vi "Eval X-Y-Z(t1,t2).vi"(0 "Start":dbl[](array[numeric])=[0.0, 0.0] format="%.2f", 1 "number of points":u32=25, 2 "End":dbl[](array[numeric])=[1.0, 1.0] format="%.2f", 3 "Formulas":string[](array[string])=["", "", ""], 4 "Variables":string[](array[string])=["t1", "t2"]) -> (5 "X":dbl[](array[numeric]) format="%.2f", 6 "Y":dbl[](array[numeric]) format="%.2f", 7 "Z":dbl[](array[numeric]) format="%.2f", 8 "ticks":u32, 9 "error":i32)   [LabVIEW 2014, in "NI_Gmath.lvlib"]
doc: "Describes a surface in 3D with two variables running over two different intervals."
uses:
  NI_Gmath.lvlib
panel:
  # "Example:\n\n number of points: 25 \n Start: 0.0 and 0.0\n End: 1.0 and 1.0\n Formulas: sin(t1*t2)+t1 and exp(t2) and -t1 \n Variables: t1 and t2"
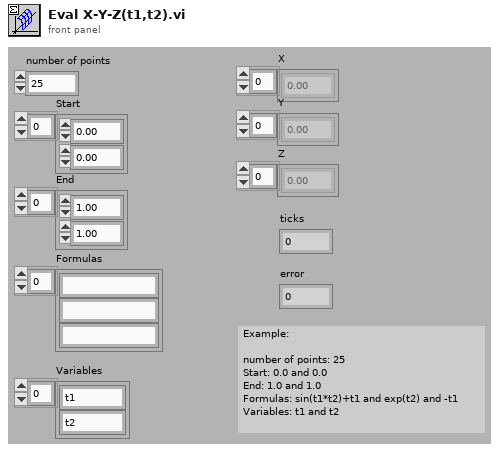
[diagram p1: front panel]
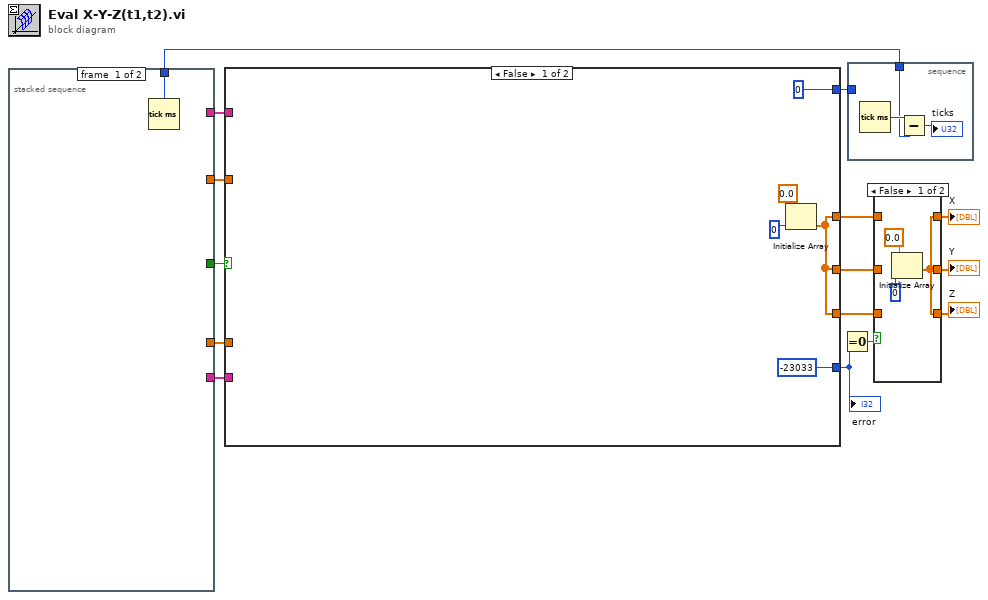
[diagram p0: block diagram]
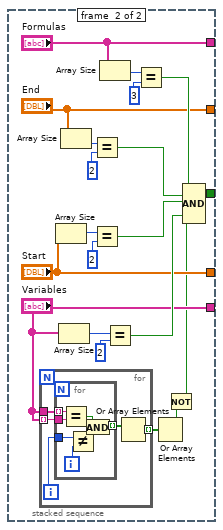
[diagram p3: hidden frame]
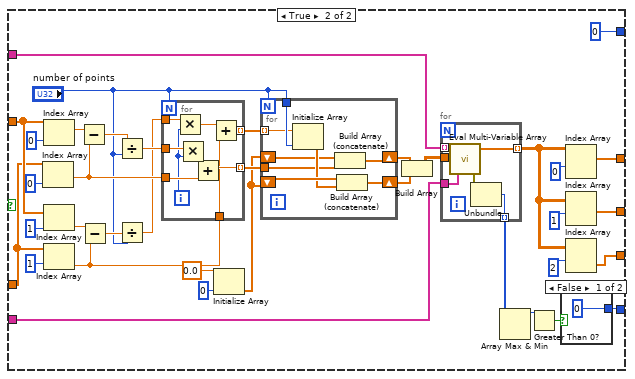
[diagram p4: hidden frame]
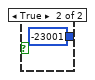
[diagram p5: hidden frame]
diagram:
  n1 = stacked-sequence {
    tunnel: [_ w36] -> w10
    tunnel: [_ "Formulas"] -> w11
    tunnel: [_ "Variables"] -> w12
    tunnel: [_ "Start"] -> w13
    tunnel: [_ "End"] -> w14
    tunnel: [w16 _] -> w9
    frame #0 {
      n2 = Tick Count (ms)() -> (millisecond timer value=w16:u32)
    }
    frame #1 {
      n3 = for {
        tunnel: "Variables" -> [w41]
        tunnel: "Variables" -> [w40] mode=indexing
        tunnel: [w37] -> w21 mode=indexing
        i -> [w39]
        n4 = for {
          tunnel: w41 -> [w48] mode=indexing
          tunnel: w40 -> [w47]
          tunnel: w39 -> [w46]
          tunnel: [w42] -> w38 mode=indexing
          i -> [w45]
          n5 = Equal?(x=w48, y=w47) -> (x = y?=w44:bool)
          n6 = Not Equal?(x=w46, y=w45) -> (x != y?=w43:bool)
          n7 = And(x=w44, y=w43) -> (x .and. y?=w42:bool)
        }
        n8 = Or Array Elements(Boolean array=w38) -> (logical OR=w37:bool)
      }
      n9 = Array Size(array="Start") -> (size(s)=w24:i32)
      n10 = Array Size(array="Variables") -> (size(s)=w28:i32)
      n11 = Array Size(array="End") -> (size(s)=w26:i32)
      n12 = Equal?(x=w26, y=2) -> (x = y?=w33:bool)
      n13 = Equal?(x=w24, y=2) -> (x = y?=w34:bool)
      n14 = Array Size(array="Formulas") -> (size(s)=w30:i32)
      n15 = Equal?(x=w28, y=2) -> (x = y?=w35:bool)
      n16 = Equal?(x=w30, y=3) -> (x = y?=w32:bool)
      n17 = Or Array Elements(Boolean array=w21) -> (logical OR=w20:bool)
      n18 = Not(x=w20) -> (.not. x?=w18:bool)
      n19 = Compound Arithmetic op=AND(w32, w33, w34, w35, w18) -> (w36:bool)
    }
  }
  n20 = case shown="False" w10 {
    tunnel: [0 0] -> w15
    tunnel: [w51 w65] -> w2
    tunnel: [w51 w64] -> w4
    tunnel: [w51 w63] -> w6
    tunnel: w14 -> [_ w62]
    tunnel: w13 -> [_ w61]
    tunnel: w11 -> [_ w60]
    tunnel: w12 -> [_ w59]
    tunnel: [-23033 w55] -> w8
    frame False {
      n21 = Initialize Array(0.0, 0) -> (w51:dbl[])
    }
    frame True {
      n22 = Index Array(array=w61, index=0) -> (element=w84:dbl)
      n23 = Index Array(array=w62, index=0) -> (element=w83:dbl)
      n24 = Index Array(array=w62, index=1) -> (element=w85:dbl)
      n25 = Index Array(array=w61, index=1) -> (element=w86:dbl)
      n26 = Subtract(x=w83, y=w84) -> (x-y=w68:dbl)
      n27 = Subtract(x=w85, y=w86) -> (x-y=w75:dbl)
      n28 = Divide(x=w68, y="number of points") -> (x/y=w78:dbl)
      n29 = Divide(x=w75, y="number of points") -> (x/y=w77:dbl)
      n30 = for {
        N: "number of points" -> [_]
        tunnel: w78 -> [w101]
        tunnel: w84 -> [w99]
        tunnel: [w98] -> w72 mode=indexing
        tunnel: w77 -> [w97]
        tunnel: w86 -> [w94]
        tunnel: [w93] -> w76 mode=indexing
        i -> [w96]
        n31 = Multiply(x=w97, y=w96) -> (x*y=w95:dbl)
        n32 = Multiply(x=w101, y=w96) -> (x*y=w100:dbl)
        n33 = Add(x=w100, y=w99) -> (x+y=w98:dbl)
        n34 = Add(x=w95, y=w94) -> (x+y=w93:dbl)
      }
      n35 = Initialize Array(0.0, 0) -> (w71:dbl[])
      n36 = for {
        N: "number of points" -> [_]
        tunnel: "number of points" -> [w109]
        tunnel: w76 -> [w108] mode=indexing
        shift-right: [w106] -> w74
        shift-left: w71 -> [w107]
        shift-right: [w104] -> w73
        shift-left: w71 -> [w103]
        tunnel: w72 -> [w102]
        n37 = Initialize Array(w108, w109) -> (w105:dbl[])
        n38 = Build Array (concatenate)(w103, w102) -> (w104:dbl[])
        n39 = Build Array (concatenate)(w107, w105) -> (w106:dbl[])
      }
      n40 = Build Array(w73, w74) -> (w87:dbl[][])
      n41 = for {
        tunnel: w59 -> [w112]
        tunnel: w60 -> [w115] mode=indexing
        tunnel: w87 -> [w113]
        tunnel: [w114] -> w66 mode=indexing
        tunnel: [w110] -> w58 mode=indexing
        n42 = call "Eval Multi-Variable Array.vi"("Variables"=w112, "X Values"=w113, "formula"=w115) -> ("error out"=w111:errorcluster, "Y Values"=w114:dbl[])  [unwired: 1 in]
        n43 = Unbundle(w111) -> ("code"=w110:i32)  [unwired: 2 out]
      }
      n44 = Array Max & Min(array=w58) -> (max value=w57:i32)  [unwired: 3 out]
      n45 = Greater Than 0?(x=w57) -> (x > 0?=w56:bool)
      n46 = case shown="False" w56 {
        tunnel: [0 -23001] -> w55
        frame False {
        }
        frame True {
        }
      }
      n47 = Index Array(array=w66, index (row)=0) -> (element=w63:dbl[])  [unwired: 1 in]
      n48 = Index Array(array=w66, index (row)=1) -> (element=w64:dbl[])  [unwired: 1 in]
      n49 = Index Array(array=w66, index (row)=2) -> (element=w65:dbl[])  [unwired: 1 in]
    }
  }
  "error" <- w8
  n50 = Equal To 0?(x=w8) -> (x = 0?=w7:bool)
  n51 = stacked-sequence {
    tunnel: w15 -> [_]
    tunnel: w9 -> [w116]
    frame #0 {
      n52 = Tick Count (ms)() -> (millisecond timer value=w118:u32)
      n53 = Subtract(x=w118, y=w116) -> (x-y=→"ticks":u32)
    }
  }
  n54 = case shown="False" w7 {
    tunnel: w6 -> [_ w124]
    tunnel: [w119 w124] -> w5
    tunnel: w4 -> [_ w123]
    tunnel: [w119 w123] -> w3
    tunnel: w2 -> [_ w122]
    tunnel: [w119 w122] -> w1
    frame False {
      n55 = Initialize Array(0.0, 0) -> (w119:dbl[])
    }
    frame True {
    }
  }
  "Y" <- w3
  "X" <- w5
  "Z" <- w1
